vi "zlock_test.vi"   [LabVIEW 2010]
types:
  T1 = typedef "zlock.ctl" = cluster{"ctx":refnum<class "zmq_context.lvclass">, "endpoint":string, "timeout":u32, "name":string}
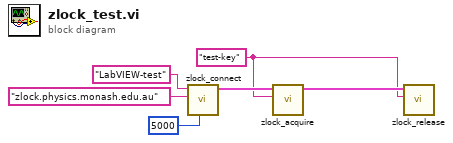
[diagram p0: block diagram]
diagram:
  w2 = "test-key" ("key")
  n1 = call <userlib>:"zlock_connect.vi"("timeout (1s)"=u32 5000, "host"="zlock.physics.monash.edu.au", "name"="LabVIEW-test") -> ("zlock"=w4:T1)  [unwired: 7 in, 1 out]
  n2 = call <userlib>:"zlock_acquire.vi"("key"=w2, "ZLock in"=w4) -> ("ZLock out"=w3:T1)  [unwired: 7 in, 2 out]
  n3 = call <userlib>:"zlock_release.vi"("key"=w2, "ZLock in"=w3) -> ()  [unwired: 7 in, 3 out]
